vi "nii_read.vi"(8 "error in (no error)":errorcluster, 11 "file (use dialog)":path) -> (0 "error out":errorcluster, 2 "data value reference":refnum<data-value>, 3 "Data":T1 {"slice orientation" items=["transverse unflipped", "coronal unflipped", "sagittal unflipped", "transverse flipped", "coronal flipped", "sagittal flipped"]}, 4 "non-flip":bool, 5 "head":u8[](array[numeric]) format="%.0x")   [LabVIEW 2014]
uses:
  control/head_data.ctl
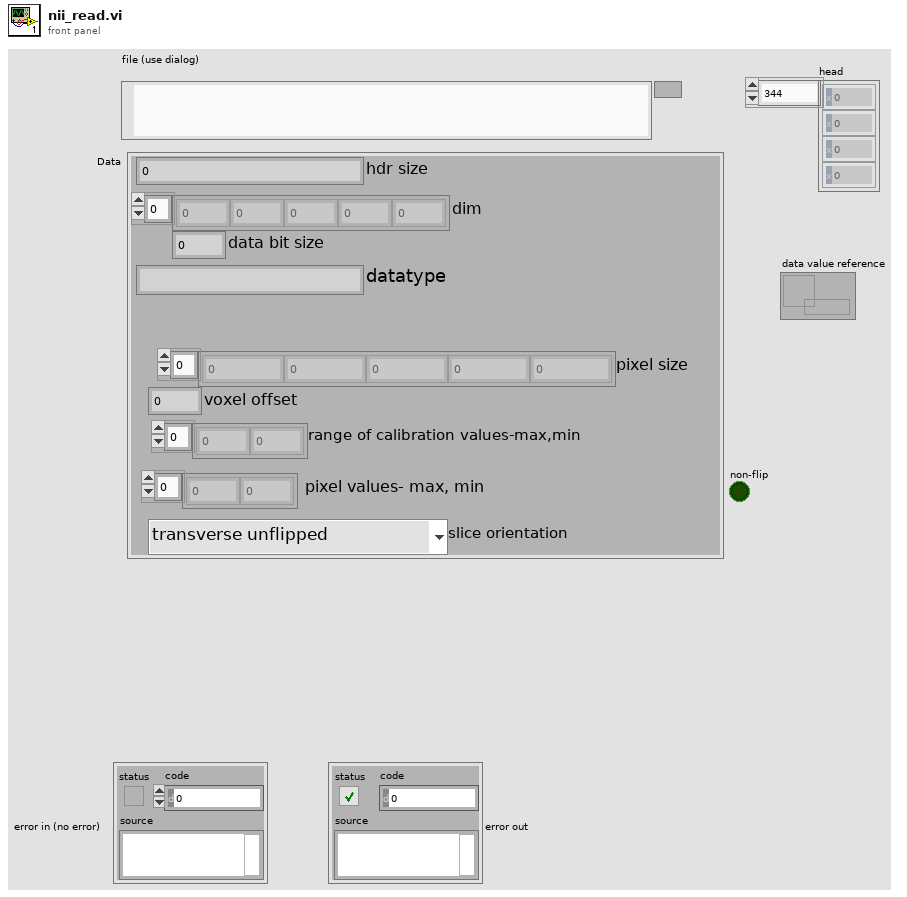
[diagram p1: front panel]
types:
  T1 = typedef "head_data.ctl" = cluster{"hdr size":i32, "dim":i32[], "data bit size":i32, "datatype":string, "pixel size ":sgl[], "voxel offset":sgl, "range of calibration values-max,min":sgl[], " pixel values- max, min":sgl[], "slice orientation":u16}
  T2 = enum16{"u_int8", "int8", "u_int16", "int16", "u_int32", "int32", "u_int64", "int64", "float", "double"}
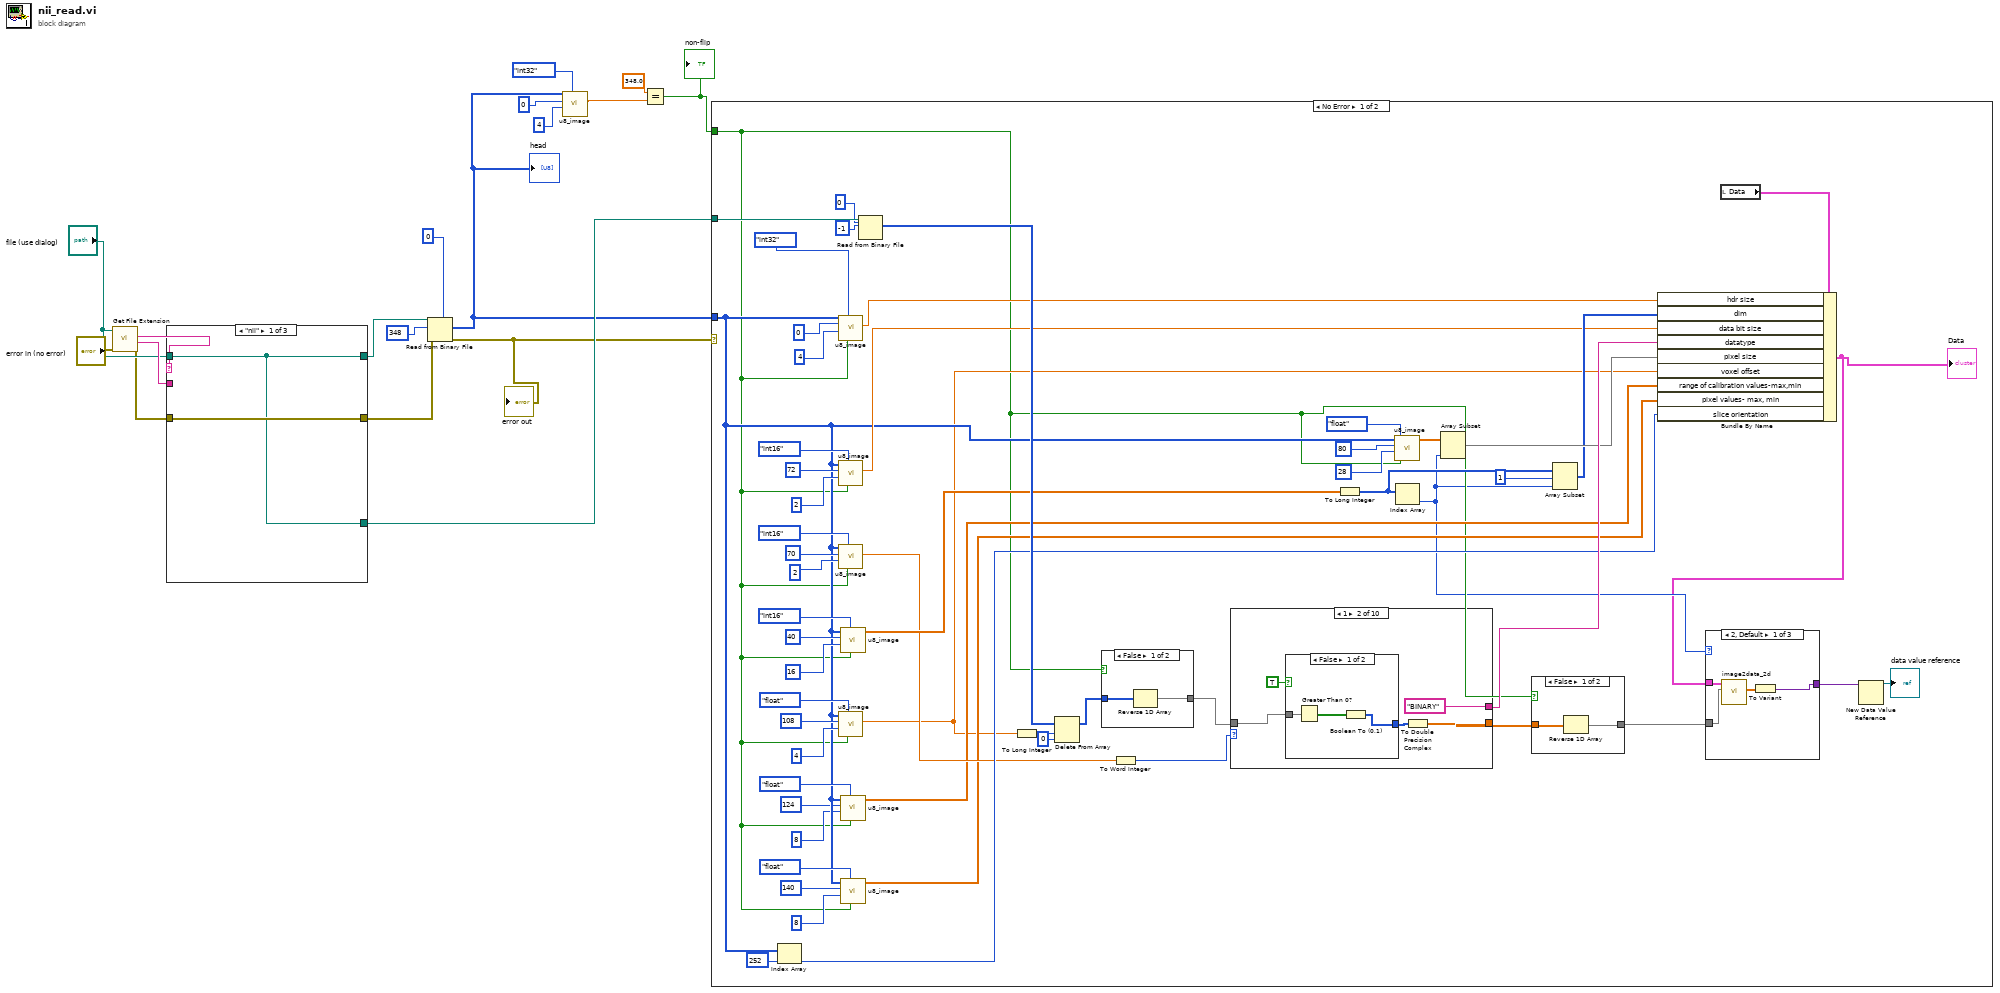
[diagram p0: block diagram]
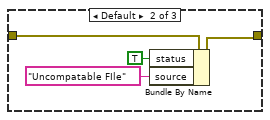
[diagram p2: hidden frame]
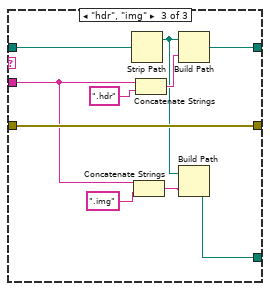
[diagram p3: hidden frame]
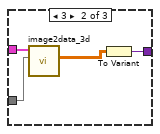
[diagram p4: hidden frame]
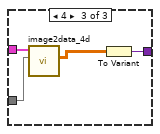
[diagram p5: hidden frame]
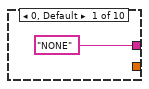
[diagram p8: hidden frame]
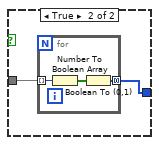
[diagram p9: hidden frame]
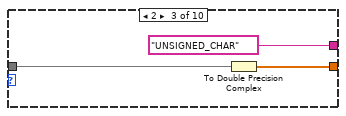
[diagram p10: hidden frame]
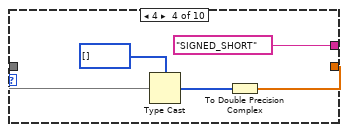
[diagram p11: hidden frame]
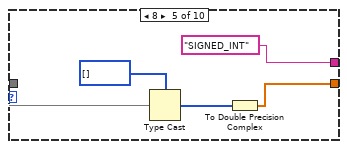
[diagram p12: hidden frame]
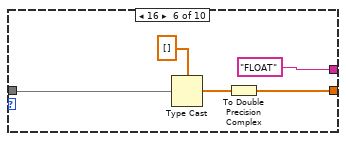
[diagram p13: hidden frame]
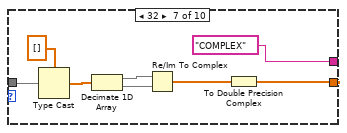
[diagram p14: hidden frame]
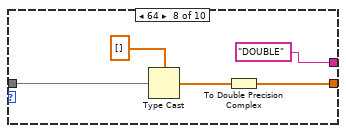
[diagram p15: hidden frame]
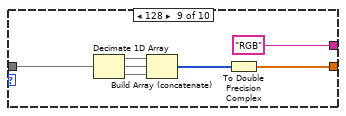
[diagram p16: hidden frame]
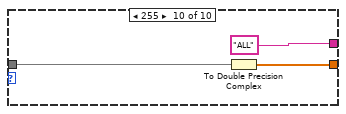
[diagram p17: hidden frame]
diagram:
  n1 = call <vilib>:"Get File Extension.vi"("error in (no error)"="error in (no error)", "file"="file (use dialog)") -> ("error out"=w14:errorcluster, "filename without extension"=w17:string, "lowercase file extension"=w18:string)  [unwired: 6 in, 1 out]
  n2 = case shown="\"nii\"" w18 {
    tunnel: "file (use dialog)" -> [w19 _ w30]
    tunnel: [w19 _ w32] -> w10
    tunnel: w17 -> [_ _ w26]
    tunnel: [w20 w23 w31] -> w15
    tunnel: w14 -> [w20 w24 w31]
    tunnel: [w19 _ w25] -> w12
    frame "nii" {
    }
    frame Default {
      n3 = Bundle By Name(cluster=w24, "status"=TRUE, "source"="Uncompatable FIle") -> (w23:errorcluster)
    }
    frame "hdr", "img" {
      n4 = Strip Path(path=w30) -> (stripped path=w29:path)  [unwired: 1 out]
      n5 = Concatenate Strings(w26, ".img" ("string")) -> (w28:string)
      n6 = Concatenate Strings(w26, ".hdr" ("string")) -> (w33:string)
      n7 = Build Path(base path=w29, name or relative path=w33) -> (appended path=w32:path)
      n8 = Build Path(base path=w29, name or relative path=w28) -> (appended path=w25:path)
    }
  }
  n9 = Read from Binary File(5:u8 0, 8:w15, 10:348 ("count (1)"), 11:w10) -> (0:w9:errorcluster, 2:w5:u8[])  [unwired: 2 in, 2 out]
  "error out" <- w9
  "head" <- w5
  n10 = call "u8_image.vi"("Enum"=T2."int32", "length"=4, "index"=0, "array"=w5) -> ("Numeric"=w3:dbl)  [unwired: 6 in, 1 out]
  n11 = Equal?(x=348.0, y=w3) -> (x = y?=w6:bool)
  "non-flip" <- w6
  n12 = case shown="No Error" w9 {
    tunnel: w5 -> [w49 _]
    tunnel: w12 -> [w91 _]
    tunnel: w6 -> [w40 _]
    frame No Error {
      n13 = Index Array(array=w49, index=252) -> (element=w83:u8)
      n14 = call "u8_image.vi"("non-flip"=w40, "Enum"=T2."int32", "length"=4, "index"=0, "array"=w49) -> ("Numeric"=w77:dbl)  [unwired: 5 in, 1 out]
      n15 = call "u8_image.vi"("non-flip"=w40, "Enum"=T2."int16", "length"=2, "index"=72, "array"=w49) -> ("Numeric"=w68:dbl)  [unwired: 5 in, 1 out]
      n16 = call "u8_image.vi"("non-flip"=w40, "Enum"=T2."int16", "length"=2, "index"=70, "array"=w49) -> ("Numeric"=w64:dbl)  [unwired: 5 in, 1 out]
      n17 = call "u8_image.vi"("non-flip"=w40, "Enum"=T2."float", "length"=4, "index"=108, "array"=w49) -> ("Numeric"=w46:dbl)  [unwired: 5 in, 1 out]
      n18 = call "u8_image.vi"("non-flip"=w40, "Enum"=T2."int16", "length"=16, "index"=40, "array"=w49) -> ("Array"=w74:dbl[])  [unwired: 5 in, 1 out]
      n19 = call "u8_image.vi"("non-flip"=w40, "Enum"=T2."float", "length"=8, "index"=124, "array"=w49) -> ("Array"=w50:dbl[])  [unwired: 5 in, 1 out]
      n20 = call "u8_image.vi"("non-flip"=w40, "Enum"=T2."float", "length"=8, "index"=140, "array"=w49) -> ("Array"=w53:dbl[])  [unwired: 5 in, 1 out]
      n21 = Read from Binary File(5:u8 0 ("default value 1"), 10:-1 ("count (1)"), 11:w91) -> (2:w88:u8[])  [unwired: 3 in, 3 out]
      n22 = To Long Integer(number=w46) -> (32bit integer=w45:i32)
      n23 = Delete From Array(array=w88, length=w45, index=0) -> (array with subset deleted=w43:u8[])  [unwired: 1 out]
      n24 = case shown="False" w40 {
        tunnel: [w107 w109] -> w42
        tunnel: w43 -> [w108 w109]
        frame False {
          n25 = Reverse 1D Array(array=w108) -> (reversed array=w107:u8[])
        }
        frame True {
        }
      }
      n26 = To Word Integer(number=w64) -> (16bit integer=w63:i16)
      n27 = case shown="1" w63 {
        tunnel: ["NONE" "BINARY" "UNSIGNED_CHAR" "SIGNED_SHORT" "SIGNED_INT" "FLOAT" "COMPLEX" "DOUBLE" "RGB" "ALL"] -> w87
        tunnel: [_ w114 w125 w130 w135 w140 w145 w153 w156 w162] -> w41
        tunnel: w42 -> [_ w113 w124 w129 w133 w137 w142 w150 w157 w163]
        frame 0, Default {
        }
        frame 1 {
          n28 = case shown="False" TRUE {
            tunnel: w113 -> [w117 w120]
            tunnel: [w116 w119] -> w112
            frame False {
              n29 = Greater Than 0?(x=w117) -> (x > 0?=w118:bool[])
              n30 = Boolean To (0,1)(Boolean=w118) -> (0, 1=w116:i16[])
            }
            frame True {
              n31 = for {
                tunnel: w120 -> [w123] mode=indexing
                tunnel: [w121] -> w119 mode=concatenating
                n32 = Number To Boolean Array(number=w123) -> (Boolean array=w122:bool[])
                n33 = Boolean To (0,1)(Boolean=w122) -> (0, 1=w121:i16[])
              }
            }
          }
          n34 = To Double Precision Complex(1:w112) -> (0:w114:cdb[])
        }
        frame 2 {
          n35 = To Double Precision Complex(1:w124) -> (0:w125:cdb[])
        }
        frame 4 {
          n36 = Type Cast(type=i16[] [], x=w129) -> (*(type *) &x=w128:i16[])
          n37 = To Double Precision Complex(1:w128) -> (0:w130:cdb[])
        }
        frame 8 {
          n38 = Type Cast(type=i32[] [], x=w133) -> (*(type *) &x=w132:i32[])
          n39 = To Double Precision Complex(1:w132) -> (0:w135:cdb[])
        }
        frame 16 {
          n40 = Type Cast(type=sgl[] [], x=w137) -> (*(type *) &x=w138:sgl[])
          n41 = To Double Precision Complex(1:w138) -> (0:w140:cdb[])
        }
        frame 32 {
          n42 = Type Cast(type=sgl[] [], x=w142) -> (*(type *) &x=w143:sgl[])
          n43 = Decimate 1D Array(w143) -> (w148:sgl[], w147:sgl[])
          n44 = Re/Im To Complex(1:w147, 2:w148) -> (0:w146:csg[])
          n45 = To Double Precision Complex(1:w146) -> (0:w145:cdb[])
        }
        frame 64 {
          n46 = Type Cast(type=dbl[] [], x=w150) -> (*(type *) &x=w151:dbl[])
          n47 = To Double Precision Complex(1:w151) -> (0:w153:cdb[])
        }
        frame 128 {
          n48 = Decimate 1D Array(w157) -> (w160:u8[], w159:u8[], w158:u8[])
          n49 = Build Array (concatenate)(w160, w159, w158) -> (w155:u8[])
          n50 = To Double Precision Complex(1:w155) -> (0:w156:cdb[])
        }
        frame 255 {
          n51 = To Double Precision Complex(1:w163) -> (0:w162:cdb[])
        }
      }
      n52 = To Long Integer(number=w74) -> (32bit integer=w80:i32[])
      n53 = call "u8_image.vi"("non-flip"=w40, "Enum"=T2."float", "length"=28, "index"=80, "array"=w49) -> ("Array"=w60:dbl[])  [unwired: 5 in, 1 out]
      n54 = Index Array(array=w80) -> (element=w39:i32)  [unwired: 1 in]
      n55 = Array Subset(array=w60, length=w39) -> (w86:dbl[])  [unwired: 1 in]
      n56 = case shown="False" w40 {
        tunnel: [w104 w106] -> w38
        tunnel: w41 -> [w105 w106]
        frame False {
          n57 = Reverse 1D Array(array=w105) -> (reversed array=w104:cdb[])
        }
        frame True {
        }
      }
      n58 = Array Subset(array=w80, index=1, length=w39) -> (w81:i32[])
      n59 = local read "Data"() -> (w85:T1)
      n60 = Bundle By Name(cluster=w85, "hdr size"=w77, "dim"=w81, "data bit size"=w68, "datatype"=w87, "pixel size"=w86, "voxel offset"=w46, "range of calibration values-max,min"=w50, "pixel values- max, min"=w53, "slice orientation"=w83) -> (w37:T1)
      "Data" <- w37
      n61 = case shown="2, Default" w39 {
        tunnel: [w95 w98 w102] -> w36
        tunnel: w37 -> [w94 w99 w103]
        tunnel: w38 -> [w93 w97 w101]
        frame 2, Default {
          n62 = call "image2data_2d.vi"("image_1d"=w93, "Data 2"=w94) -> ("imag2_2d"=w92:dbl[][])  [unwired: 8 in, 1 out]
          n63 = To Variant(anything=w92) -> (Variant=w95:variant)
        }
        frame 3 {
          n64 = call "image2data_3d.vi"("image_1d"=w97, "Data 2"=w99) -> ("imag3_3d"=w96:dbl[][][])  [unwired: 8 in, 1 out]
          n65 = To Variant(anything=w96) -> (Variant=w98:variant)
        }
        frame 4 {
          n66 = call "image2data_4d.vi"("image_1d"=w101, "Data"=w103) -> ("image_4d"=w100:dbl[][][][])  [unwired: 8 in, 1 out]
          n67 = To Variant(anything=w100) -> (Variant=w102:variant)
        }
      }
      n68 = New Data Value Reference(data value=w36) -> (data value reference=→"data value reference":refnum<data-value>)  [unwired: 1 in, 1 out]
    }
    frame Error {
    }
  }
